vi "test_pearson_map.vi"() -> ()   [LabVIEW 2009]
doc: "Copyright (C) 2009, Stepan A. Baranov\nweb: http://www.OCTLab.org/\nemail: stepan@baranov.su"
uses:
  OCTLib.dll
  <vilib>/gmath/NI_Gmath.lvlib
panel:
  out "version":string
  out "name":string
  out "error out":errorcluster
  out "cell height":i32
  out "cell width":i32
  out "A-scan size":i32
  out "# of A-scans":i32
  in  "Small/Big":bool
  out "loop #":i32
  out "RSM_STAT time":u32
  out "LabView time":u32
  out "RSM_STAT Array":dbl[][](array[numeric])
  out "LabView Array":dbl[][](array[numeric])
  in  "stop":bool
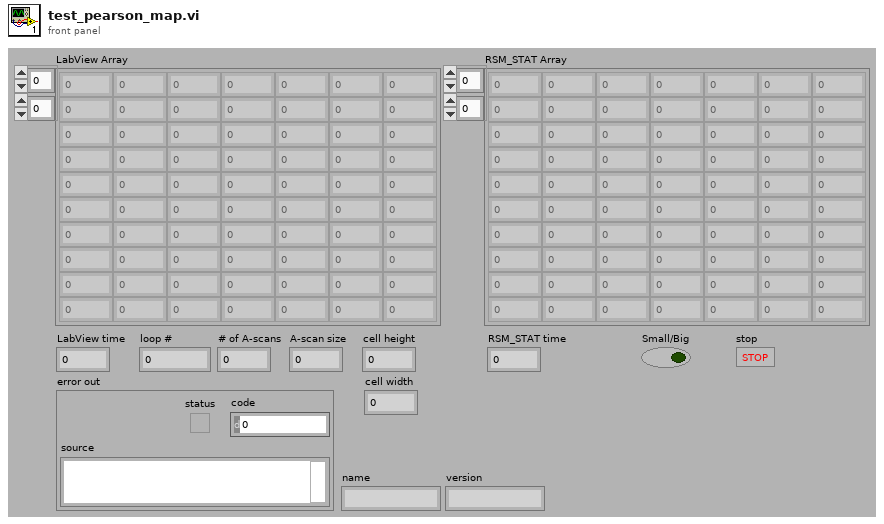
[diagram p1: front panel]
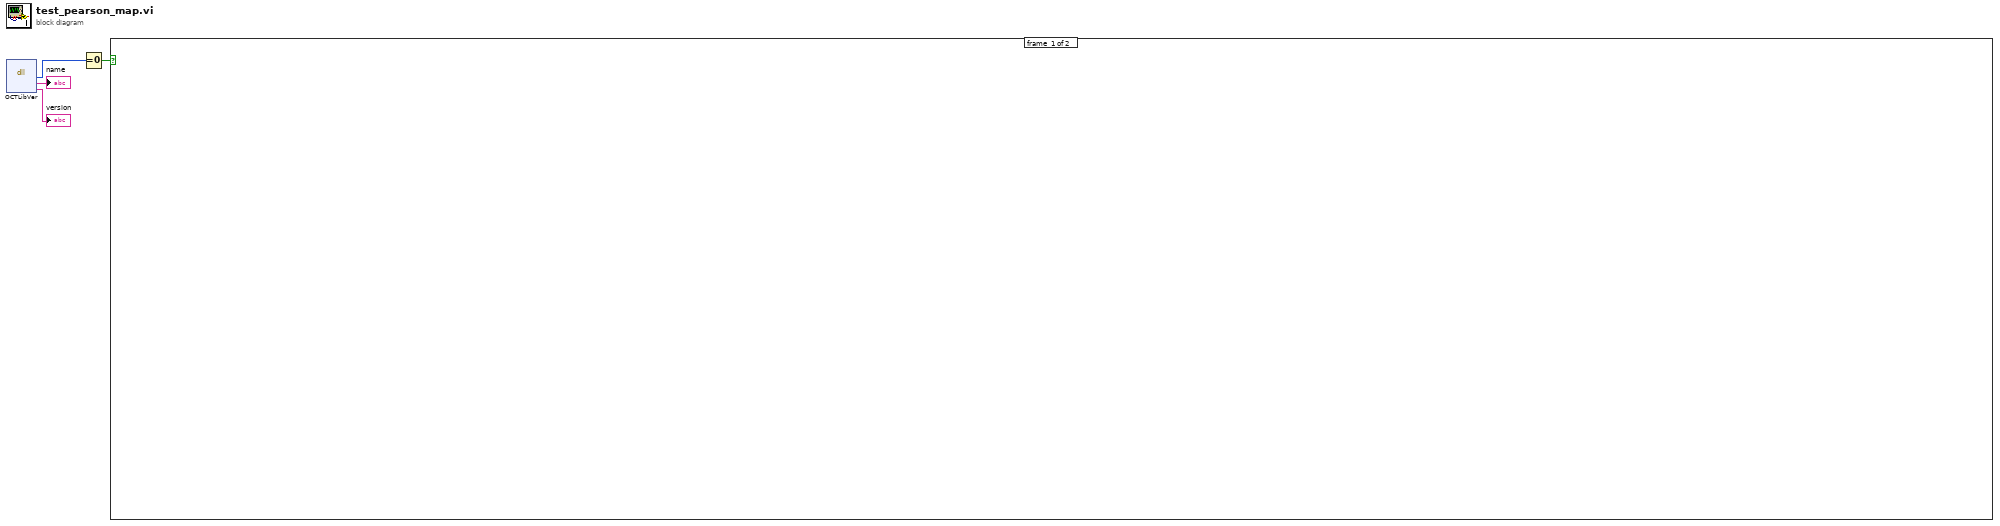
[diagram p0: block diagram]
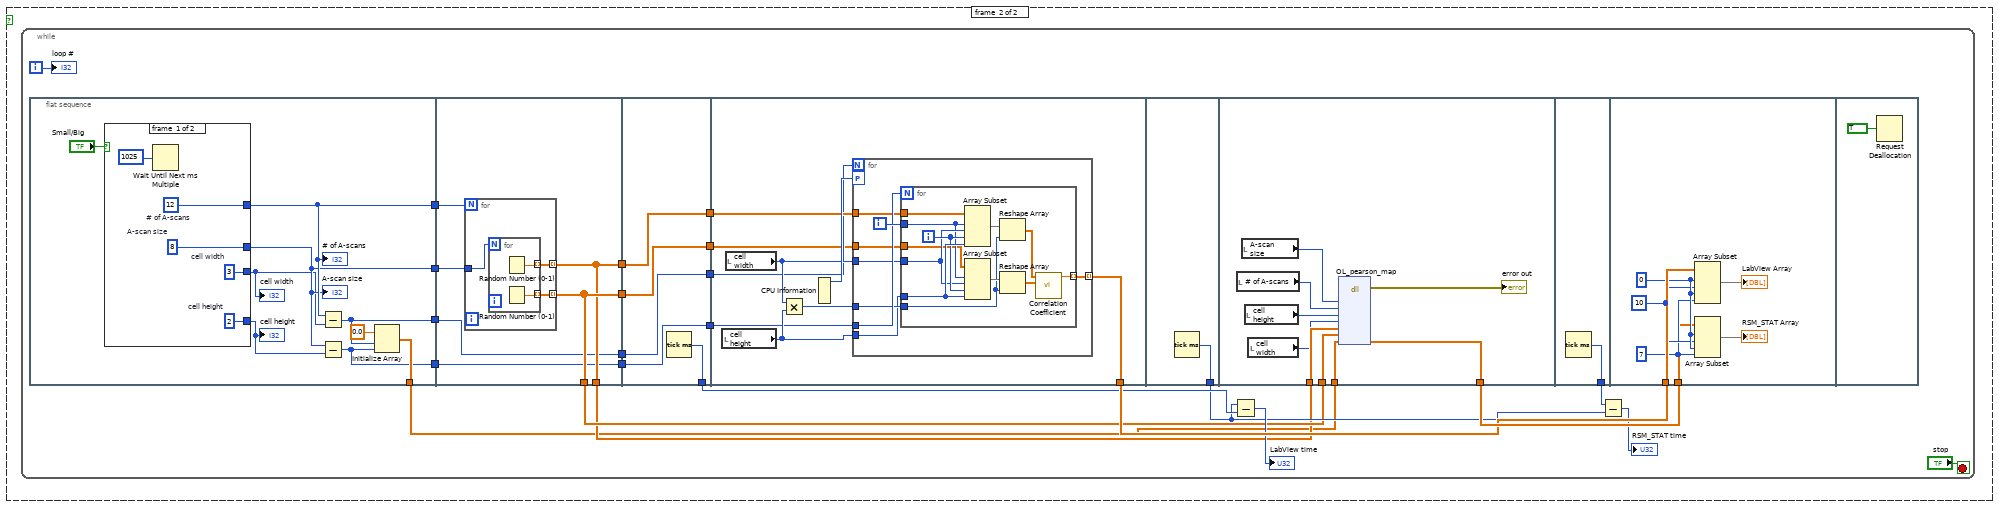
[diagram p2: hidden frame]
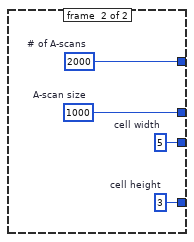
[diagram p3: hidden frame]
diagram:
  n1 = dll-call lib="OCTLib.dll" fn="OCTLibVer"() -> ("status"=w4:i8, "name"=→"name":string, "version"=→"version":string)  [unwired: 5 in, 2 out]
  n2 = Equal To 0?(x=w4) -> (x = 0?=w3:bool)
  n3 = case shown="True" w3 {
    frame #0 {
    }
    frame #1 {
      n4 = while {
        i -> [w20]
        stop <- "stop" stop-if-true
        n5 = flat-sequence {
          tunnel: [w34] -> w16
          tunnel: [w36] -> w15
          tunnel: [w33] -> w11
          tunnel: [w30] -> w7
          tunnel: [w29] -> w5
          tunnel: [w52] -> w19
          tunnel: [w52] -> w17
          tunnel: w16 -> [w50]
          tunnel: w15 -> [w49]
          tunnel: [w51] -> w14
          tunnel: [w51] -> w12
          tunnel: [w47] -> w9
          tunnel: w7 -> [w48]
          tunnel: [w48] -> w6
          tunnel: w5 -> [w47]
          tunnel: [w62] -> w25
          tunnel: [w61] -> w18
          tunnel: w17 -> [w61]
          tunnel: w14 -> [w60]
          tunnel: [w60] -> w13
          tunnel: [w59] -> w10
          tunnel: w9 -> [w59]
          tunnel: [w58] -> w8
          tunnel: w6 -> [w58]
          tunnel: [w64] -> w26
          tunnel: w18 -> [w63]
          tunnel: w13 -> [w67]
          tunnel: w10 -> [w66]
          tunnel: w8 -> [w65]
          tunnel: [w92] -> w22
          tunnel: w19 -> [w98]
          tunnel: [w101] -> w27
          tunnel: w12 -> [w97]
          tunnel: w11 -> [w94]
          tunnel: [w102] -> w23
          tunnel: w27 -> [w103]
          tunnel: w26 -> [w109]
          frame #0 {
            n6 = case shown="False" "Small/Big" {
              tunnel: [w41 w45] -> w36
              tunnel: [w42 w46] -> w34
              tunnel: [w39 w44] -> w31
              tunnel: [w38 w43] -> w32
              frame #0 {
                w38 = 2  # cell height
                w39 = 3  # cell width
                w42 = 8  # A-scan size
                w41 = 12  # # of A-scans
                n7 = Wait Until Next ms Multiple(millisecond multiple=u32 1025) -> ()  [unwired: 1 out]
              }
              frame #1 {
                w43 = 3  # cell height
                w44 = 5  # cell width
                w46 = 1000  # A-scan size
                w45 = 2000  # # of A-scans
              }
            }
            "# of A-scans" <- w36
            "A-scan size" <- w34
            "cell width" <- w31
            "cell height" <- w32
            n8 = Subtract(x=w36, y=w31) -> (x-y=w30:i32)
            n9 = Subtract(x=w34, y=w32) -> (x-y=w29:i32)
            n10 = Initialize Array(0.0 ("element"), w30, w29) -> (w33:dbl[][])
          }
          frame #1 {
            n11 = for {
              N: w49 -> [_]
              tunnel: w50 -> [w55]
              tunnel: [w54] -> w52 mode=indexing
              tunnel: [w53] -> w51 mode=indexing
              n12 = for {
                N: w55 -> [_]
                tunnel: [w57] -> w54 mode=indexing
                tunnel: [w56] -> w53 mode=indexing
                n13 = Random Number (0-1)() -> (number: 0 to 1=w56:dbl)
                n14 = Random Number (0-1)() -> (number: 0 to 1=w57:dbl)
              }
            }
          }
          frame #2 {
            n15 = Tick Count (ms)() -> (millisecond timer value=w62:u32)
          }
          frame #3 {
            n16 = local read "cell height"() -> (w69:i32)
            n17 = local read "cell width"() -> (w70:i32)
            n18 = Multiply(x=w70, y=w69) -> (x*y=w68:i32)
            n19 = CPU Information() -> (4:w71:i32)  [unwired: 3 out]
            n20 = for {
              N: w65 -> [_]
              tunnel: [w78] -> w64 mode=indexing
              workers-P: w71 -> [_]
              tunnel: w66 -> [w77]
              tunnel: w68 -> [w76]
              tunnel: w70 -> [w75]
              tunnel: w69 -> [w74]
              tunnel: w67 -> [w73]
              tunnel: w63 -> [w72]
              i -> [w79]
              n21 = for {
                N: w77 -> [_]
                tunnel: w79 -> [w86]
                tunnel: [w80] -> w78 mode=indexing
                tunnel: w76 -> [w83]
                tunnel: w75 -> [w87]
                tunnel: w74 -> [w89]
                tunnel: w73 -> [w90]
                tunnel: w72 -> [w85]
                i -> [w88]
                n22 = Array Subset(array=w90, index (row)=w86, length (row)=w87, index (col)=w88, length (col)=w89) -> (w91:dbl[][])
                n23 = Array Subset(array=w85, index (row)=w86, length (row)=w87, index (col)=w88, length (col)=w89) -> (w84:dbl[][])
                n24 = Reshape Array(w91, w83) -> (w81:dbl[])
                n25 = Reshape Array(w84, w83) -> (w82:dbl[])
                n26 = call <vilib>:"Correlation Coefficient.vi"("Y"=w82, "X"=w81) -> ("correlation coefficient r"=w80:dbl)  [unwired: 8 in, 1 out]
              }
            }
          }
          frame #4 {
            n27 = Tick Count (ms)() -> (millisecond timer value=w92:u32)
          }
          frame #5 {
            n28 = local read "# of A-scans"() -> (w99:i32)
            n29 = local read "A-scan size"() -> (w100:i32)
            n30 = local read "cell height"() -> (w96:i32)
            n31 = local read "cell width"() -> (w95:i32)
            n32 = dll-call lib="OCTLib.dll" fn="OL_pearson_map"("A-scan size"=w100, "# of A-scan"=w99, "cell height"=w96, "cell width"=w95, "input1"=w97, "input2"=w98, "data"=w94) -> (error out=→"error out":errorcluster, "data"=w101:dbl[][])  [unwired: 10 in, 1 out]
          }
          frame #6 {
            n33 = Tick Count (ms)() -> (millisecond timer value=w102:u32)
          }
          frame #7 {
            w106 = 10 ("length")
            w105 = 7 ("length")
            w107 = 0 ("index")
            n34 = Array Subset(array=w109, index (row)=w107, length (row)=w106, index (col)=w107, length (col)=w105) -> (→"LabView Array":dbl[][])
            n35 = Array Subset(array=w103, index (row)=w107, length (row)=w106, index (col)=w107, length (col)=w105) -> (→"RSM_STAT Array":dbl[][])
          }
          frame #8 {
            n36 = Request Deallocation(TRUE ("flag")) -> ()
          }
        }
        n37 = Subtract(x=w22, y=w25) -> (x-y=→"LabView time":u32)
        n38 = Subtract(x=w23, y=w22) -> (x-y=→"RSM_STAT time":u32)
        "loop #" <- w20
      }
    }
  }
